vi "TwTpsSetActiveFilament.vi"(1 "activeFilament":i32, 2 "error in (no error)":errorcluster) -> (0 "error out":errorcluster)   [LabVIEW 2009]
uses:
  TofDaqDll.dll
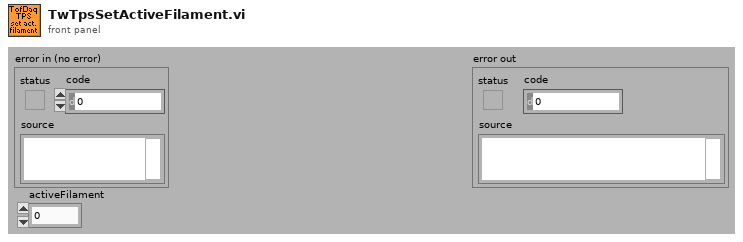
[diagram p1: front panel]
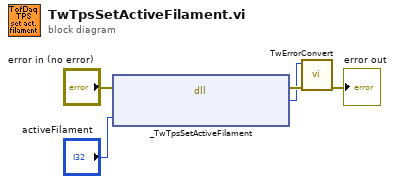
[diagram p0: block diagram]
diagram:
  n1 = dll-call lib="C:/src/TofDaq/APIandWrappers/LabView/TofDaqDll/TofDaqDll.dll" fn="_TwTpsSetActiveFilament"(error in="error in (no error)", "activeFilament"="activeFilament") -> (error out=w4:errorcluster, "TwRetVal"=w2:i32)  [unwired: 2 in, 2 out]
  n2 = call "TwErrorConvert.vi"("error in (no error)"=w4, "error code"=w2) -> ("error out"=→"error out":errorcluster)  [unwired: 9 out]
